vi "CPTR Align Math.vi"(6 "sync.cptr.period":u16=1, 8 "error in":errorcluster, 10 "measured cptr adjust distance":u16, 11 "sync.cptr.adjust":u16=1) -> (0 "error out":errorcluster, 3 "new cptr adjust":u16)   [LabVIEW 2012, in "ni579x Synchronization v1 Host.lvlib"]
doc: "Based on the input measurement and current CPTR Adjust amount, compute the new CPTR Adjust amount. This VI will handle wrap-around incase the new adjust is greater than the CPTR period. This VI will also check that the new CPTR Adjust is within the valid range of [0, CPTR Period) and error if it is not."
uses:
  <instrlib>/ni579x/Synchronization/v1/Host/ni579x Synchronization v1 Host.lvlib
  <vilib>/ErrorRing/Error Ring.xnode
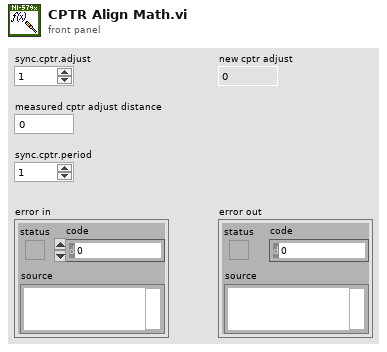
[diagram p1: front panel]
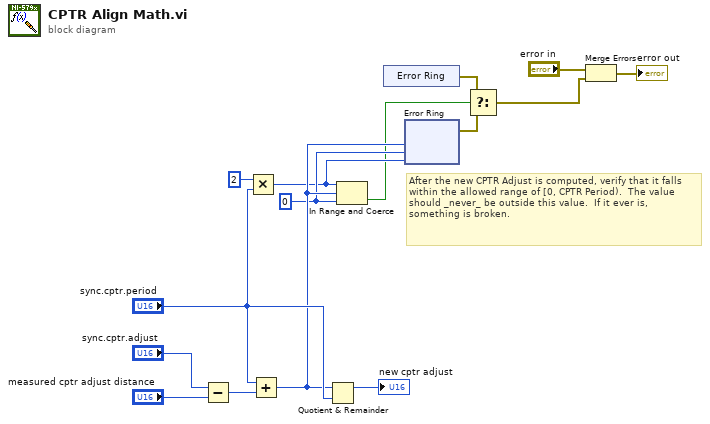
[diagram p0: block diagram]
diagram:
  w3 = 0 ("lower limit")
  # "After the new CPTR Adjust is computed, verify that it falls within the allowed range of [0, CPTR Period).  The value should _never_ be outside this value.  If it ever is, something is broken."
  n1 = Subtract(x="sync.cptr.adjust", y="measured cptr adjust distance") -> (x-y=w13:i32)
  n2 = Multiply(x=2 ("y"), y="sync.cptr.period") -> (x*y=w2:i32)
  n3 = Add(x="sync.cptr.period", y=w13) -> (x+y=w4:i32)
  n4 = Quotient & Remainder(x=w4, y="sync.cptr.period") -> (x-y*floor(x/y)=→"new cptr adjust":i32)  [unwired: 1 out]
  n5 = In Range and Coerce(upper limit=w2, x=w4, lower limit=w3) -> (In Range?=w1:bool)  [unwired: 1 out]
  n6 = xnode "Error Ring"() -> ("error out"=w9:errorcluster)
  n7 = xnode "Error Ring"("parameter 0"=w4, "parameter 1"=w3, "parameter 2"=w2) -> ("error out"=w8:errorcluster)
  n8 = Select(t=w9, s=w1, f=w8) -> (s? t:f=w7:errorcluster)
  n9 = Merge Errors("error in", w7) -> (→"error out":errorcluster)
